vi "Config Data Modify.vi"(0 "config data":T3, 1 "function":T2=enum."put data", 2 "section":string, 3 "key":string, 5 "destroy (F)":bool, 7 "file path":path, 9 "section names":string[](array[string]), 11 "error in (no error)":errorcluster, 12 "data":T1[](array[typedef]), 13 "value":string) -> (4 "config data out":T3, 6 "section exists?":bool, 8 "key exists?":bool, 15 "error out":errorcluster)   [LabVIEW 2009]
doc: "Modifies data associated with an object. All functions that want get the data, operate on it, and set the data, should go through this VI in order to avoid race conditions."
uses:
  <vilib>/Utility/config.llb/Config Data RefNum.ctl
  Config Data Modify Functions.ctl
  Config Data Section.ctl
  Config Data Registry Functions.ctl
  <vilib>/Utility/config.llb/NI_LVConfig.lvlib
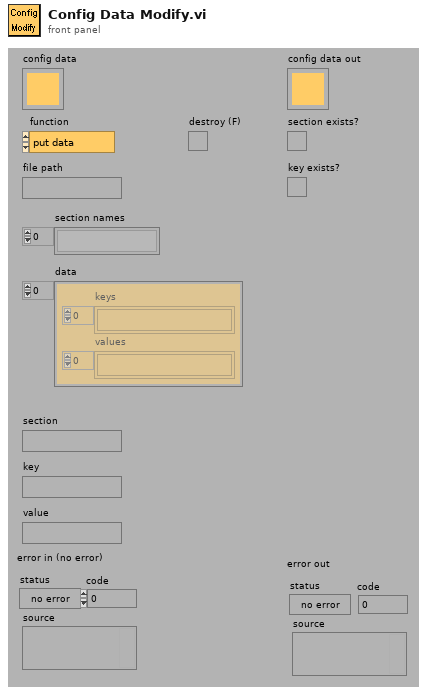
[diagram p1: front panel]
types:
  T1 = typedef "Config Data Section.ctl" = cluster{"keys":string[], "values":string[]}
  T2 = typedef "Config Data Modify Functions.ctl" = enum16{"set file path", "put data", "add key", "remove section", "remove key"}
  T3 = typedef "NI_LVConfig.lvlib/Config Data RefNum.ctl" = refnum<k1>
  T4 = typedef "Config Data Registry Functions.ctl" = enum16{"reset", "register", "get data", "get section", "set data", "unregister", "test", "get objects"}
  T5 = typedef "Config Data.ctl" = cluster{"file path":path, "data":T1[], "section names":string[]}
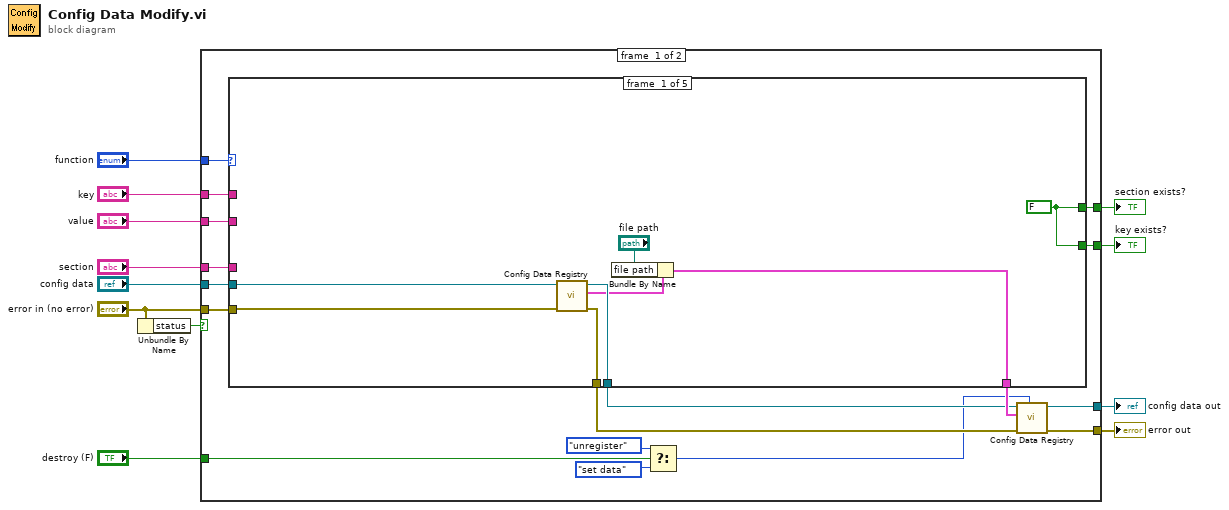
[diagram p0: block diagram]
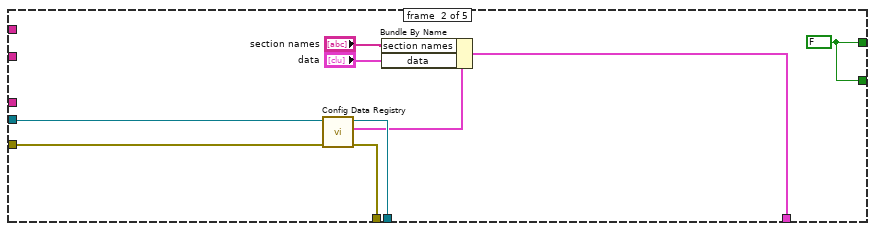
[diagram p2: hidden frame]
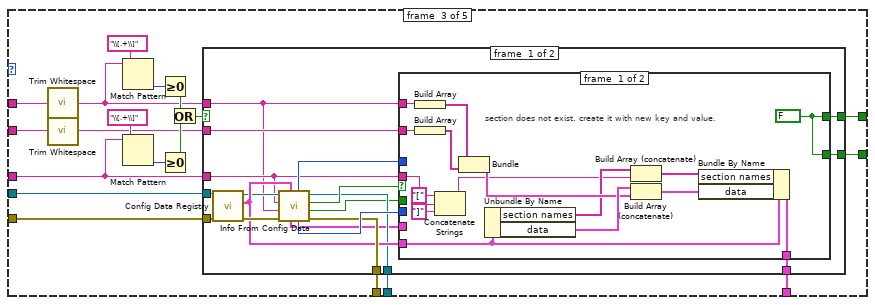
[diagram p3: hidden frame]
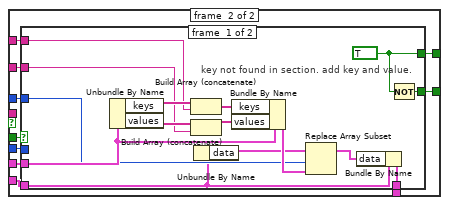
[diagram p4: hidden frame]
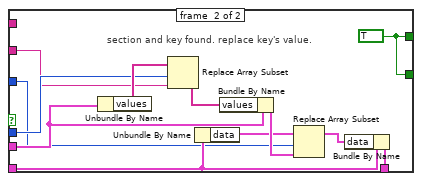
[diagram p5: hidden frame]
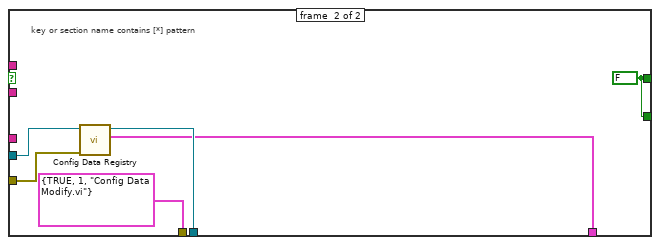
[diagram p6: hidden frame]
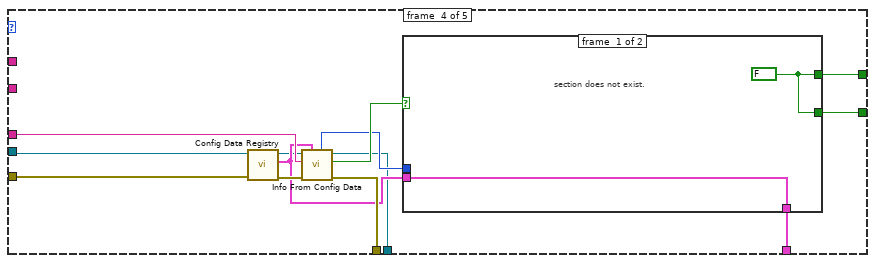
[diagram p7: hidden frame]
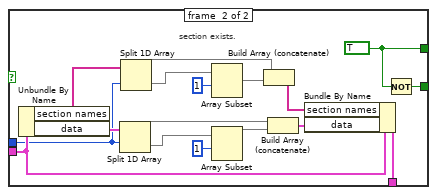
[diagram p8: hidden frame]
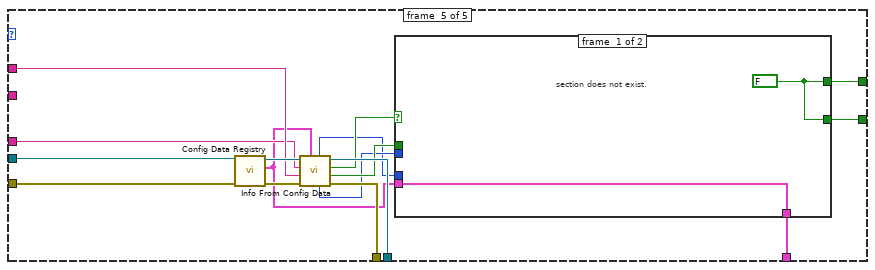
[diagram p9: hidden frame]
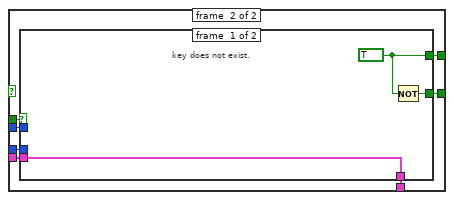
[diagram p10: hidden frame]
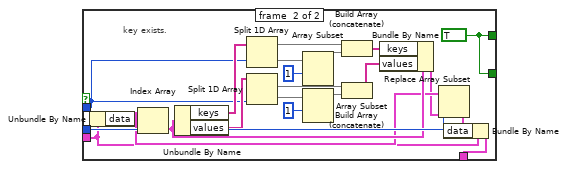
[diagram p11: hidden frame]
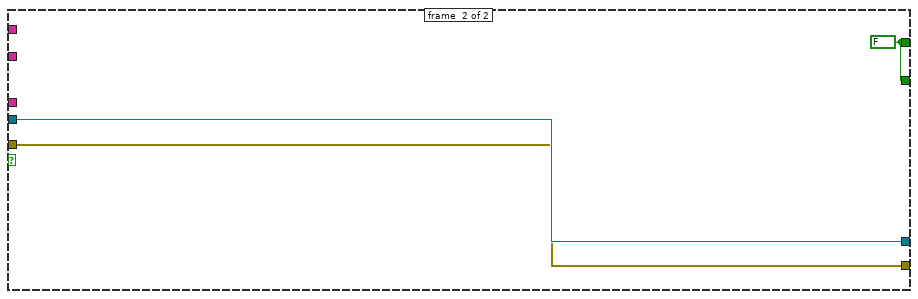
[diagram p12: hidden frame]
diagram:
  n1 = Unbundle By Name("error in (no error)") -> ("status"=w1:bool)
  n2 = case shown="False" w1 {
    tunnel: "error in (no error)" -> [w16 w225]
    tunnel: [w29 w225] -> w12
    tunnel: "config data" -> [w18 w226]
    tunnel: [w28 w226] -> w10
    tunnel: "function" -> [w27 _]
    tunnel: "destroy (F)" -> [w26 _]
    tunnel: "key" -> [w24 _]
    tunnel: "value" -> [w23 _]
    tunnel: "section" -> [w22 _]
    tunnel: [w21 w224] -> w4
    tunnel: [w20 w224] -> w3
    frame #0 {
      n3 = case shown="\"add key\"" w27 {
        tunnel: [w37 w46 w65 w155 w190] -> w25
        tunnel: [w33 w44 w59 w143 w182] -> w19
        tunnel: w22 -> [_ _ w52 w148 w179]
        tunnel: w23 -> [_ _ w48 _ _]
        tunnel: w24 -> [_ _ w50 _ w180]
        tunnel: [w35 w45 w64 w154 w189] -> w21
        tunnel: [w35 w45 w63 w153 w188] -> w20
        tunnel: w18 -> [w34 w40 w61 w151 w186]
        tunnel: [w32 w43 w60 w149 w183] -> w17
        tunnel: w16 -> [w30 w41 w62 w152 w187]
        frame #0 {
          w35 = FALSE
          n4 = call "Config Data Registry.vi"("error in (no error)"=w30, "config data"=w34) -> ("error out"=w32:errorcluster, 2:"config data out"=w31:T5, 3:"config data out"=w33:T3)  [unwired: 3 in, 4 out]
          n5 = Bundle By Name(cluster=w31, "file path"="file path") -> (w37:T5)
        }
        frame #1 {
          w45 = FALSE
          n6 = call "Config Data Registry.vi"("error in (no error)"=w41, "config data"=w40) -> ("error out"=w43:errorcluster, 2:"config data out"=w42:T5, 3:"config data out"=w44:T3)  [unwired: 3 in, 4 out]
          n7 = Bundle By Name(cluster=w42, "section names"="section names", "data"="data") -> (w46:T5)
        }
        frame #2 {
          n8 = call <vilib>:"Trim Whitespace.vi"("string"=w50) -> ("trimmed string"=w49:string)  [unwired: 1 in]
          n9 = call <vilib>:"Trim Whitespace.vi"("string"=w48) -> ("trimmed string"=w47:string)  [unwired: 1 in]
          n10 = Match Pattern(string=w49, regular expression="\\[.+\\]") -> (offset past match=w56:i32)  [unwired: 1 in, 3 out]
          n11 = Match Pattern(string=w52, regular expression="\\[.+\\]") -> (offset past match=w55:i32)  [unwired: 1 in, 3 out]
          n12 = Greater Or Equal To 0?(x=w56) -> (x >= 0?=w54:bool)
          n13 = Greater Or Equal To 0?(x=w55) -> (x >= 0?=w53:bool)
          n14 = Or(x=w54, y=w53) -> (x .or. y?=w51:bool)
          n15 = case shown="False" w51 {
            tunnel: [w83 w138] -> w65
            tunnel: [w82 w137] -> w64
            tunnel: [w81 w137] -> w63
            tunnel: w62 -> [w80 w140]
            tunnel: w61 -> [w79 w141]
            tunnel: w47 -> [w78 _]
            tunnel: [w75 cluster{bool, u16, string} {TRUE, 1, "Config Data Modify.vi"}] -> w60
            tunnel: [w71 w139] -> w59
            tunnel: w52 -> [w67 _]
            tunnel: w49 -> [w66 _]
            frame #0 {
              n16 = call "Config Data Registry.vi"("error in (no error)"=w80, "config data"=w79) -> ("error out"=w76:errorcluster, 2:"config data out"=w74:T5, 3:"config data out"=w73:T3)  [unwired: 3 in, 4 out]
              n17 = call "Info From Config Data.vi"("config data in"=w74, "error in (no error)"=w76, "key"=w66, "section"=w67, "config data"=w73) -> ("error out"=w75:errorcluster, "key exists?"=w69:bool, "section exists?"=w72:bool, "config data out"=w71:T3, "key index"=w77:i32, "section index"=w68:i32, "section contents"=w70:T1)
              n18 = case shown="True" w72 {
                tunnel: w70 -> [_ w108]
                tunnel: w67 -> [w89 _]
                tunnel: w66 -> [w99 w107]
                tunnel: w78 -> [w98 w106]
                tunnel: [w95 w105] -> w83
                tunnel: w69 -> [_ w109]
                tunnel: [w91 w104] -> w82
                tunnel: [w91 w103] -> w81
                tunnel: w74 -> [w90 w102]
                tunnel: w77 -> [_ w101]
                tunnel: w68 -> [_ w100]
                frame #0 {
                  w91 = FALSE
                  # "section does not exist. create it with new key and value."
                  n19 = Build Array(w99) -> (w96:string[])
                  n20 = Build Array(w98) -> (w97:string[])
                  n21 = Concatenate Strings("[", w89, "]") -> (w85:string)
                  n22 = Bundle(w96, w97) -> (w93:cluster{string[], string[]})  [unwired: 1 in]
                  n23 = Unbundle By Name(w90) -> ("section names"=w86:string[], "data"=w94:T1[])
                  n24 = Build Array (concatenate)(w86, w85) -> (w84:string[])
                  n25 = Build Array (concatenate)(w94, w93) -> (w92:T1[])
                  n26 = Bundle By Name(cluster=w90, "section names"=w84, "data"=w92) -> (w95:T5)
                }
                frame #1 {
                  n27 = case shown="True" w109 {
                    tunnel: w108 -> [w114 w128]
                    tunnel: w107 -> [w122 _]
                    tunnel: w106 -> [w121 w131]
                    tunnel: [w113 w134] -> w105
                    tunnel: w101 -> [_ w132]
                    tunnel: [w116 w129] -> w104
                    tunnel: [w115 w129] -> w103
                    tunnel: w102 -> [w111 w127]
                    tunnel: w100 -> [w112 w125]
                    frame #0 {
                      w116 = TRUE
                      # "key not found in section. add key and value."
                      n28 = Unbundle By Name(w114) -> ("keys"=w124:string[], "values"=w123:string[])
                      n29 = Build Array (concatenate)(w124, w122) -> (w120:string[])
                      n30 = Build Array (concatenate)(w123, w121) -> (w119:string[])
                      n31 = Unbundle By Name(w111) -> ("data"=w110:T1[])
                      n32 = Bundle By Name(cluster=w114, "keys"=w120, "values"=w119) -> (w118:T1)
                      n33 = Replace Array Subset(array=w110, new element=w118, index=w112) -> (w117:T1[])
                      n34 = Bundle By Name(cluster=w111, "data"=w117) -> (w113:T5)
                      n35 = Not(x=w116) -> (.not. x?=w115:bool)
                    }
                    frame #1 {
                      w129 = TRUE
                      # "section and key found. replace key's value."
                      n36 = Unbundle By Name(w128) -> ("values"=w133:string[])
                      n37 = Replace Array Subset(array=w133, new element=w131, index=w132) -> (w130:string[])
                      n38 = Unbundle By Name(w127) -> ("data"=w126:T1[])
                      n39 = Bundle By Name(cluster=w128, "values"=w130) -> (w136:T1)
                      n40 = Replace Array Subset(array=w126, new element=w136, index=w125) -> (w135:T1[])
                      n41 = Bundle By Name(cluster=w127, "data"=w135) -> (w134:T5)
                    }
                  }
                }
              }
            }
            frame #1 {
              w137 = FALSE
              # "key or section name contains [*] pattern"
              n42 = call "Config Data Registry.vi"("error in (no error)"=w140, "config data"=w141) -> (2:"config data out"=w138:T5, 3:"config data out"=w139:T3)  [unwired: 3 in, 5 out]
            }
          }
        }
        frame #3 {
          n43 = call "Config Data Registry.vi"("error in (no error)"=w152, "config data"=w151) -> ("error out"=w150:errorcluster, 2:"config data out"=w147:T5, 3:"config data out"=w146:T3)  [unwired: 3 in, 4 out]
          n44 = call "Info From Config Data.vi"("config data in"=w147, "error in (no error)"=w150, "section"=w148, "config data"=w146) -> ("error out"=w149:errorcluster, "section exists?"=w145:bool, "config data out"=w143:T3, "section index"=w144:i32)  [unwired: 1 in, 3 out]
          n45 = case shown="True" w145 {
            tunnel: [w157 w168] -> w155
            tunnel: w147 -> [w157 w169]
            tunnel: w144 -> [_ w159]
            tunnel: [w156 w166] -> w154
            tunnel: [w156 w165] -> w153
            frame #0 {
              w156 = FALSE
              # "section does not exist."
            }
            frame #1 {
              w166 = TRUE
              # "section exists."
              n46 = Unbundle By Name(w169) -> ("section names"=w160:string[], "data"=w174:T1[])
              n47 = Split 1D Array(array=w174, index=w159) -> (first subarray=w170:T1[], second subarray=w173:T1[])
              n48 = Split 1D Array(array=w160, index=w159) -> (first subarray=w162:string[], second subarray=w163:string[])
              n49 = Array Subset(array=w163, index=1) -> (w161:string[])  [unwired: 1 in]
              n50 = Array Subset(array=w173, index=1) -> (w171:T1[])  [unwired: 1 in]
              n51 = Build Array (concatenate)(w162, w161) -> (w158:string[])
              n52 = Build Array (concatenate)(w170, w171) -> (w167:T1[])
              n53 = Bundle By Name(cluster=w169, "section names"=w158, "data"=w167) -> (w168:T5)
              n54 = Not(x=w166) -> (.not. x?=w165:bool)
            }
          }
        }
        frame #4 {
          n55 = call "Config Data Registry.vi"("error in (no error)"=w187, "config data"=w186) -> ("error out"=w185:errorcluster, 2:"config data out"=w178:T5, 3:"config data out"=w184:T3)  [unwired: 3 in, 4 out]
          n56 = call "Info From Config Data.vi"("config data in"=w178, "error in (no error)"=w185, "key"=w180, "section"=w179, "config data"=w184) -> ("error out"=w183:errorcluster, "key exists?"=w177:bool, "section exists?"=w181:bool, "config data out"=w182:T3, "key index"=w176:i32, "section index"=w175:i32)  [unwired: 1 out]
          n57 = case shown="True" w181 {
            tunnel: w178 -> [w192 w199]
            tunnel: [w192 w198] -> w190
            tunnel: w175 -> [_ w197]
            tunnel: w176 -> [_ w196]
            tunnel: [w191 w195] -> w189
            tunnel: [w191 w194] -> w188
            tunnel: w177 -> [_ w193]
            frame #0 {
              w191 = FALSE
              # "section does not exist."
            }
            frame #1 {
              n58 = case shown="True" w193 {
                tunnel: [w202 w204] -> w198
                tunnel: w199 -> [w202 w206]
                tunnel: w197 -> [_ w223]
                tunnel: w196 -> [_ w220]
                tunnel: [w201 w203] -> w195
                tunnel: [w200 w203] -> w194
                frame #0 {
                  w201 = TRUE
                  # "key does not exist."
                  n59 = Not(x=w201) -> (.not. x?=w200:bool)
                }
                frame #1 {
                  w203 = TRUE
                  # "key exists."
                  n60 = Unbundle By Name(w206) -> ("data"=w208:T1[])
                  n61 = Index Array(array=w208, index=w223) -> (element=w211:T1)
                  n62 = Unbundle By Name(w211) -> ("keys"=w222:string[], "values"=w221:string[])
                  n63 = Split 1D Array(array=w222, index=w220) -> (first subarray=w213:string[], second subarray=w217:string[])
                  n64 = Split 1D Array(array=w221, index=w220) -> (first subarray=w214:string[], second subarray=w216:string[])
                  n65 = Array Subset(array=w217, index=1) -> (w212:string[])  [unwired: 1 in]
                  n66 = Array Subset(array=w216, index=1) -> (w215:string[])  [unwired: 1 in]
                  n67 = Build Array (concatenate)(w213, w212) -> (w210:string[])
                  n68 = Build Array (concatenate)(w214, w215) -> (w209:string[])
                  n69 = Bundle By Name(cluster=w211, "keys"=w210, "values"=w209) -> (w207:T1)
                  n70 = Replace Array Subset(array=w208, new element=w207, index=w223) -> (w205:T1[])
                  n71 = Bundle By Name(cluster=w206, "data"=w205) -> (w204:T5)
                }
              }
            }
          }
        }
      }
      n72 = Select(t=Config_Data_Registry_Functions."unregister" ("function (get data)"), s=w26, f=Config_Data_Registry_Functions."set data" ("function (get data)")) -> (s? t:f=w13:T4)
      n73 = call "Config Data Registry.vi"("function (get data)"=w13, "error in (no error)"=w17, "config data in"=w25, "config data"=w19) -> ("error out"=w29:errorcluster, "config data out"=w28:T3)  [unwired: 1 in, 5 out]
    }
    frame #1 {
      w224 = FALSE
    }
  }
  "config data out" <- w10
  "error out" <- w12
  "section exists?" <- w4
  "key exists?" <- w3
